vi "Get User VI Application Instance.vi"(8 "error in":errorcluster, 11 "User VI Ref":refnum<vi>) -> (0 "error out":errorcluster, 1 "VI Of Top-Most Block Diagram":string, 2 "Application Name":string, 3 "User VI Application Instance Ref":refnum<vi>, 4 "This Application Reference":u32)   [LabVIEW 2022 SP3]
doc: "<add documentation here>"
panel:
  # "Development\nControls or indicators that are useful for development or testing, but which are not outputs of the VI."
  # "Input\nInputs to the VI"
  # "Output\nOutputs of the VI"
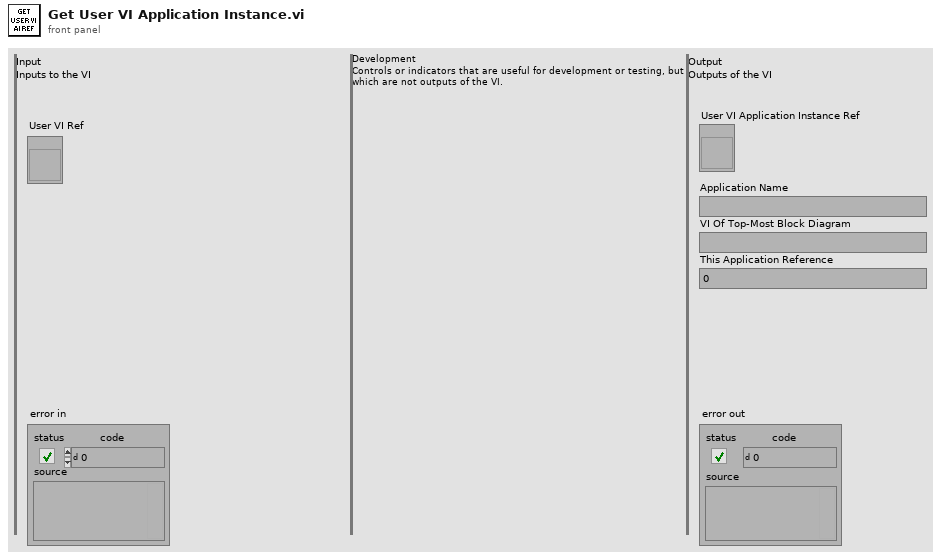
[diagram p1: front panel]
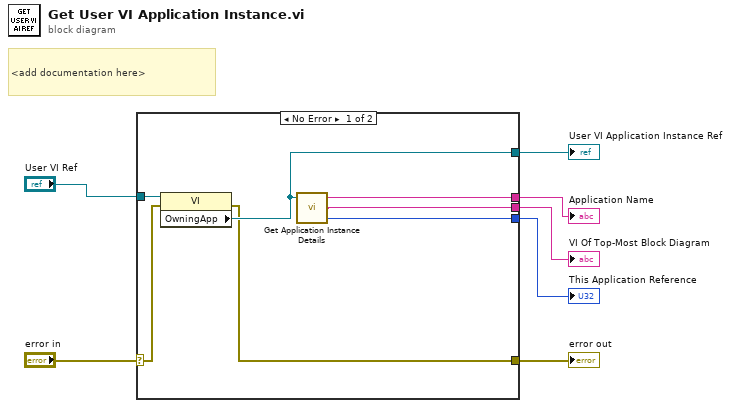
[diagram p0: block diagram]
diagram:
  # "<add documentation here>"
  n1 = case shown="No Error" "error in" {
    selector: "error in" -> [w9 w15]
    tunnel: "User VI Ref" -> [w14 _]
    tunnel: [w13 _] -> w6
    tunnel: [w12 _] -> w5
    tunnel: [w11 _] -> w4
    tunnel: [w10 _] -> w3
    tunnel: [w8 w15] -> w1
    frame No Error {
      n2 = property class="VI"(reference=w14, error in=w9) -> (error out=w8:errorcluster, "OwningApp"=w13:refnum<vi>)  [unwired: 1 out]
      n3 = call "Get Application Instance Details.vi"("Application Instance Ref"=w13) -> ("This Application Reference"=w10:u32, "VI Of Top-Most Block Diagram"=w11:string, "Application Name"=w12:string)  [unwired: 2 in]
    }
    frame Error {
    }
  }
  "Application Name" <- w5
  "VI Of Top-Most Block Diagram" <- w4
  "This Application Reference" <- w3
  "User VI Application Instance Ref" <- w6
  "error out" <- w1
